vi "ExperimentCode_Serial.vi"() -> ()   [LabVIEW 2017]
uses:
  <vilib>/Analysis/baseanly.llb/Mean (DBL).vi
  <vilib>/Instr/_visa.llb/VISA Configure Serial Port (Instr).vi
  <vilib>/express/express shared/transition.llb/Dynamic To Waveform Array.vi
  <vilib>/express/express signal manip/GetorSetDDTAttributes/Set DDT Attributes/SetT0.vi
  <vilib>/express/express shared/transition.llb/Waveform Array To Dynamic.vi
  <vilib>/express/express signal manip/GetorSetDDTAttributes/Set DDT Attributes/Set DDT Properties.xnode
  <vilib>/Analysis/NI_AALBase.lvlib
panel:
  in  "Tab Control":enum32{"Setup ", "Experiment Controls", "Debug"}(tab)=enum."Experiment Controls"
  in  "Max Torque":dbl=21.3
  in  "Servo 1 Zero Offset":dbl=-4.0
  in  "Servo 2 Zero Offset":dbl=1.0
  in  "Servo 3 Zero Offset":dbl=7.0
  in  "Servo 4 Zero Offset":dbl
  in  "Servo 5 Zero Offset":dbl
  in  "Servo 5 Torque Intercept":dbl
  in  "Servo 5 Torque Slope":dbl=1.0
  in  "Servo 5 Position Intercept":dbl
  in  "Servo 5 Position Slope":dbl=1.0
  in  "Servo 4 Torque Intercept":dbl
  in  "Servo 4 Torque Slope":dbl=1.0
  in  "Servo 4 Position Intercept":dbl
  in  "Servo 4 Position Slope":dbl=1.0
  in  "Servo 3 Torque Intercept":dbl=-72.1928
  in  "Servo 3 Torque Slope":dbl=0.002332
  in  "Servo 3 Position Intercept":dbl=111.82
  in  "Servo 3 Position Slope":dbl=-0.00449
  in  "Servo 2 Torque Intercept":dbl=-72.1928
  in  "Servo 2 Torque Slope":dbl=0.002332
  in  "Servo 2 Position Intercept":dbl=97.9723
  in  "Servo 2 Position Slope":dbl=-0.00488
  in  "Servo 1 Torque Intercept":dbl=-72.1928
  in  "Servo 1 Torque Slope":dbl=0.002332
  in  "Servo 1 Position Intercept":dbl
  in  "Servo 1 Position Slope":dbl=-0.004988
  in  "Plot Last x Seconds":dbl=100.0
  in  "COM Port":refnum<visa-resource-name>
  in  "Buad Rate":i32(ring)=115200 items=["2400"=2400, "4800"=4800, "9600"=9600, "14400"=14400, "19200"=19200, "28800"=28800, "38400"=38400, "57600"=57600, "115200"=115200]
  in  "Lowest Servo Angle":dbl=-65.0
  in  "Highest Servo Angle":dbl=65.0
  in  "Number of Servos":dbl=3.0
  out "Maximum Torque Exceeded":bool
  in  "Save":bool
  in  "Stop VI":bool
  in  "Sample Frequency":dbl=100.0 step=50.0
  out "Servo Torque":cluster{" Time Offset":dbl, dbl, dbl[][]}(graph)
  in  "Tail Amplitude (cm)":dbl=2.0
  in  "Length of Segments":dbl=10.0
  in  "Number of Waves":dbl=1.0
  in  "Wave Exponential":dbl=2.0
  in  "Frequency":dbl=1.0
  in  "Wave Form":u16(ring) items=["Sine", "Exponentional Sine", "Second Mode Bending", "Flat Plate"]
  in  "Wind Up Waveform":bool
  in  "Mode 1 Amplitude":dbl=0.1 step=0.1
  in  "Mode 2 Amplitude":dbl=0.2 step=0.1
  in  "Mode 1 Phase":dbl step=0.1
  in  "Mode 2 Phase":dbl=0.8499 step=0.1
  in  "Wind Down Waveform":bool
  in  "Wind Down Time":i32=5
  out "Waveform":cluster{"X Nodes":dbl[], "Y Nodes":dbl[]}[](graph)
  in  "Servo Input":bool
  in  "Send Waveform to MBE":bool
  in  "Servo 5 Input":dbl
  in  "Servo 4 Input":dbl
  in  "Servo 3 Input":dbl
  in  "Servo 2 Input":dbl
  in  "Servo 1  Input":dbl
  out "Minimum or Maximum Angle Exceeded":bool
  in  "Filename":path=path "test.tdms"
  in  "Comment":string
  out "Calculated Sample Frequency":dbl
  out "Specified Time Delay":dbl
  out "Calculated Time Delay":dbl
  out "Time Elapsed":dbl
  out "Output Angles":dbl[](array[numeric])
  out "Input Angles":dbl[](array[numeric])
  out "Pos5 number":dbl
  out "Pos4 number":dbl
  out "Pos3 number":dbl
  out "Pos2 number":dbl
  out "Pos1 number":dbl
  out "Torq1 number":dbl
  out "Torq2 number":dbl
  out "Torq3 number":dbl
  out "Torq4 number":dbl
  out "Torq5 number":dbl
  out "Servo 1 Position":cluster{" Time Offset":dbl, "mean":dbl, dbl[][]}(graph)
  out "Servo 2 Position":cluster{" Time Offset":dbl, "mean":dbl, dbl[][]}(graph)
  out "Servo 3 Position":cluster{" Time Offset":dbl, "mean":dbl, dbl[][]}(graph)
  out "Servo 4 Position":cluster{" Time Offset":dbl, "mean":dbl, dbl[][]}(graph)
  out "Servo 5 Position":cluster{" Time Offset":dbl, "mean":dbl, dbl[][]}(graph)
  out "Sent to Arduino":string
  out "Bytes at port":cluster{i32, dbl, dbl[]}(graph)
  out "Read Buffer":string
  # "deg"
  # "deg"
  # "deg"
  # "deg"
  # "deg"
  # "Waveform"
  # "Manual"
  # "cm"
  # "Hz"
  # "Off"
  # "On"
  # "rad"
  # "rad"
  # "Off"
  # "On"
  # "Hz"
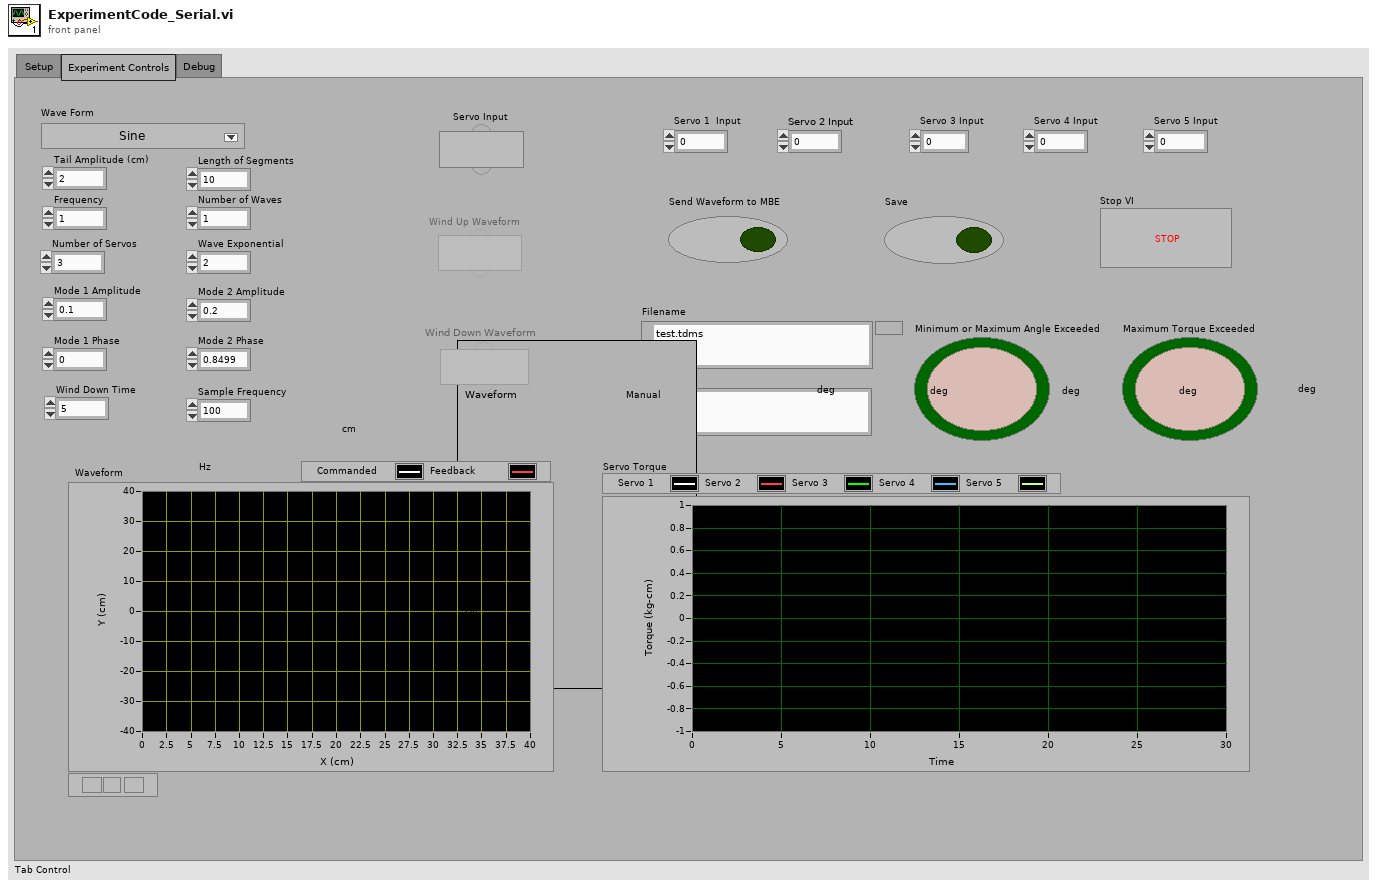
[diagram p1: front panel]
types:
  T1 = enum8{"Enabled", "Disabled", "Disabled and Grayed Out"}
  T2 = cluster{"Tail Amplitude (cm)":dbl, "Frequency":dbl, "Number of Waves":dbl, "Length of Segments":dbl, "Wave Exponential":dbl, "Number of Servos":dbl, "Mode 1 Amplitude":dbl, "Mode 2 Amplitude":dbl, "Mode 1 Phase":dbl, "Mode 2 Phase":dbl}
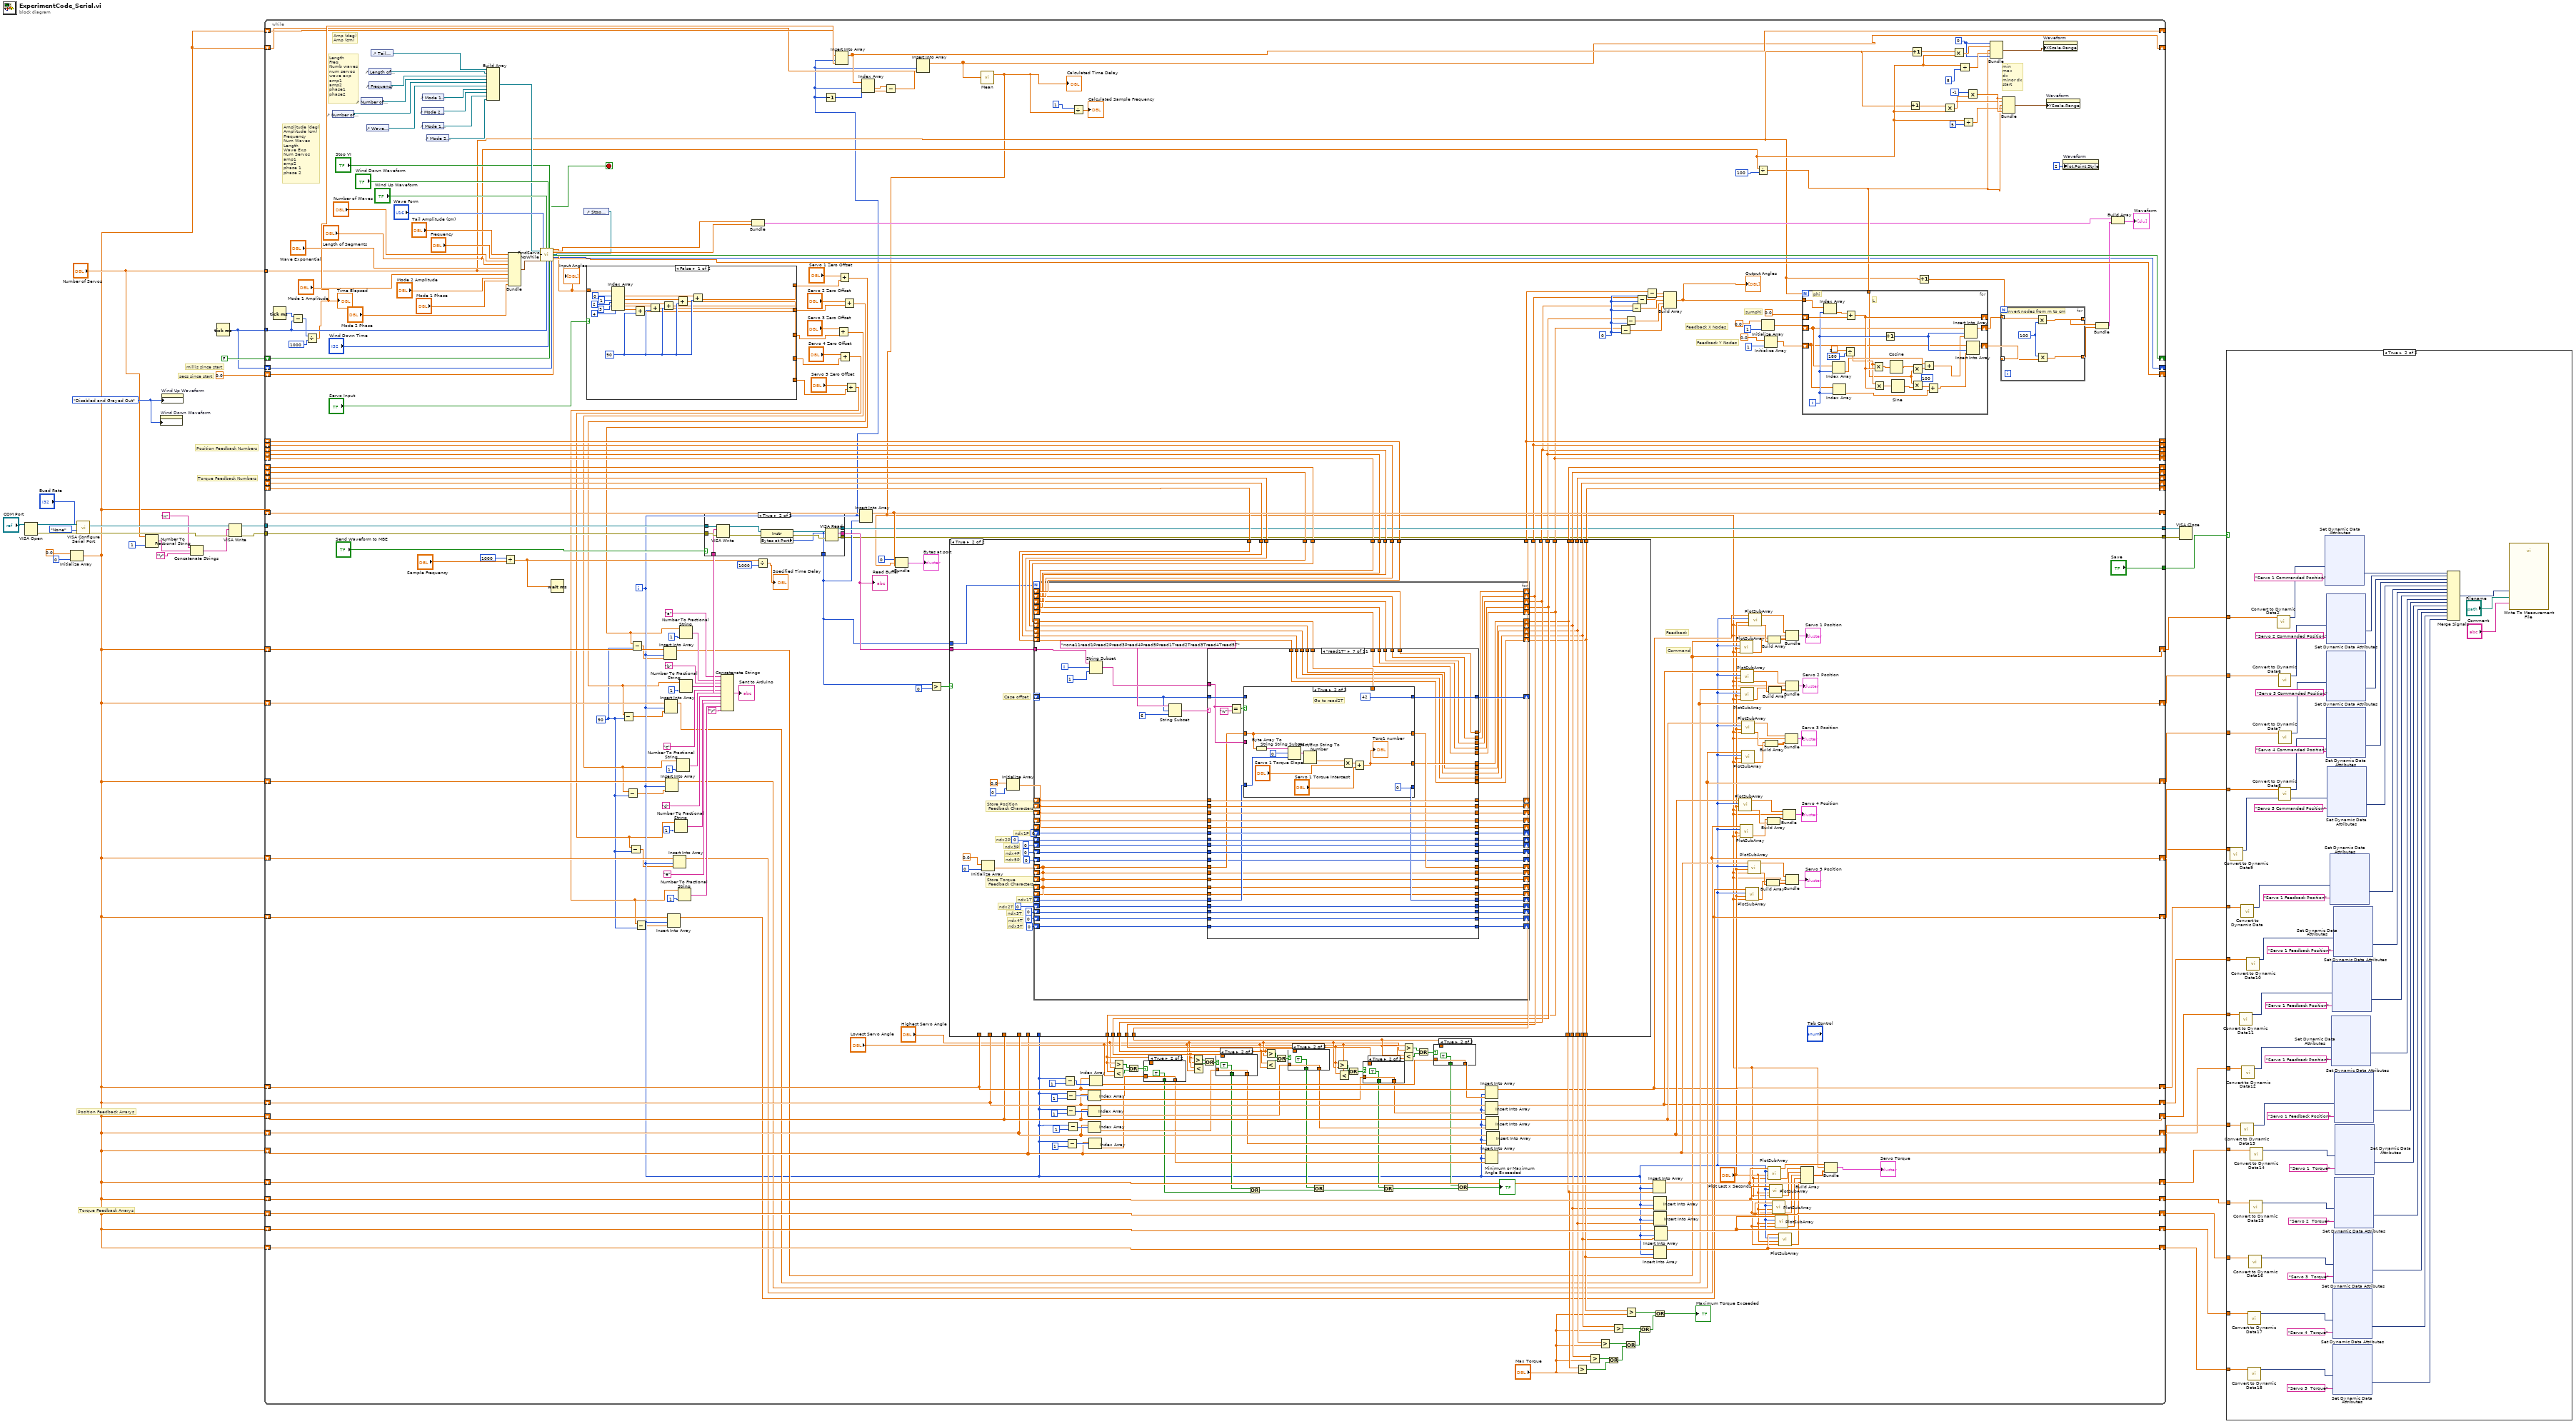
[diagram p0: block diagram]
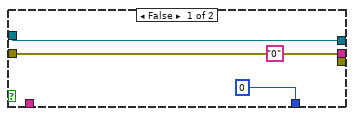
[diagram p3: hidden frame]
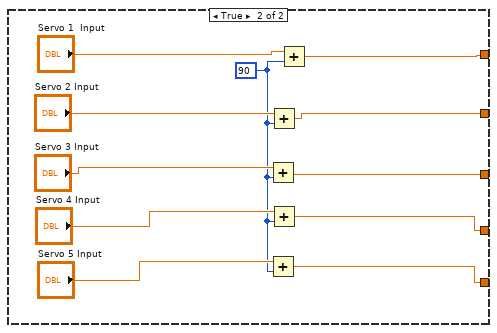
[diagram p4: hidden frame]
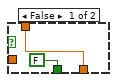
[diagram p5: hidden frame]
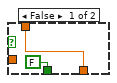
[diagram p6: hidden frame]
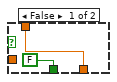
[diagram p7: hidden frame]
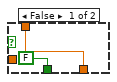
[diagram p8: hidden frame]
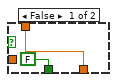
[diagram p9: hidden frame]
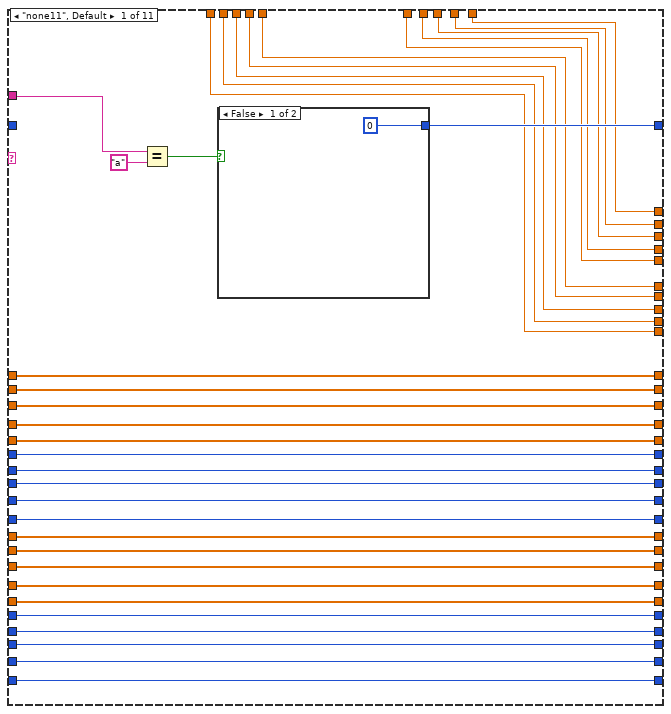
[diagram p11: hidden frame]
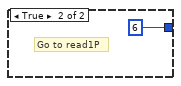
[diagram p12: hidden frame]
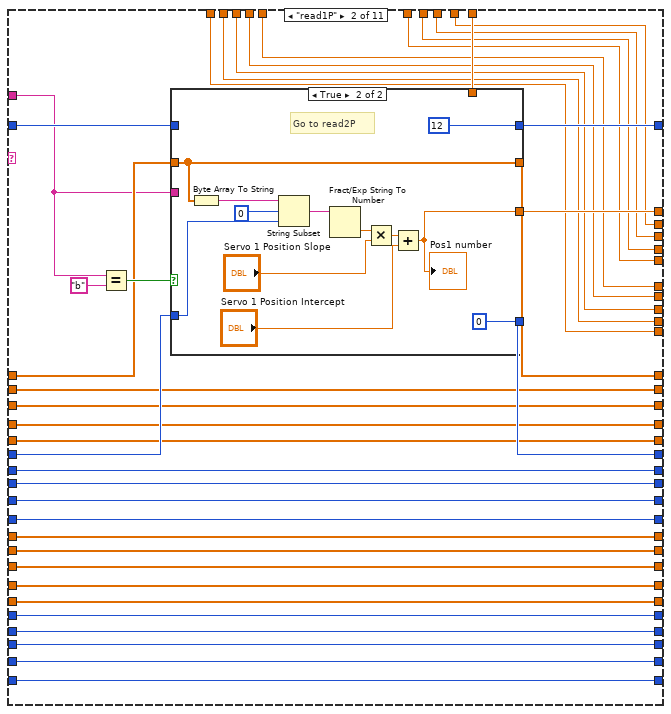
[diagram p13: hidden frame]
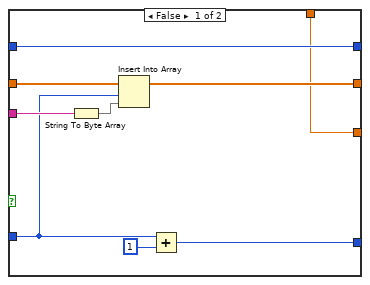
[diagram p14: hidden frame]
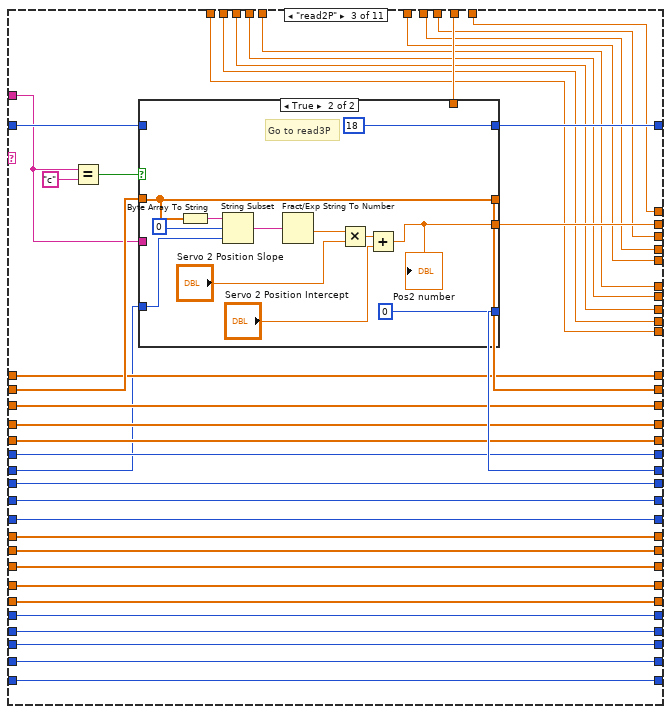
[diagram p15: hidden frame]
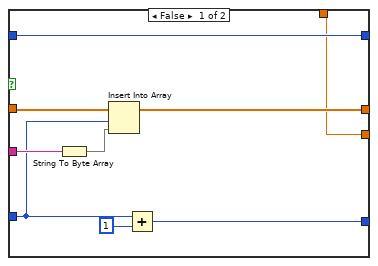
[diagram p16: hidden frame]
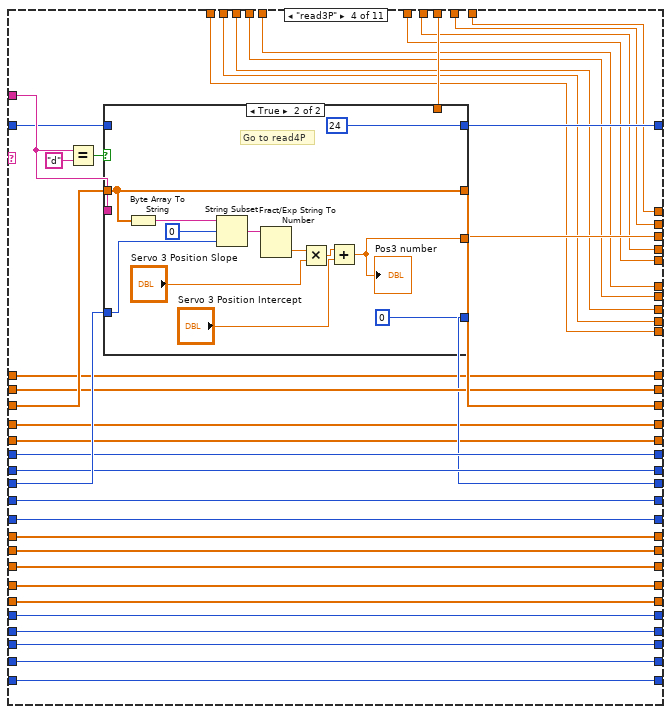
[diagram p17: hidden frame]
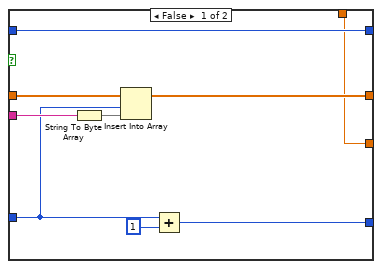
[diagram p18: hidden frame]
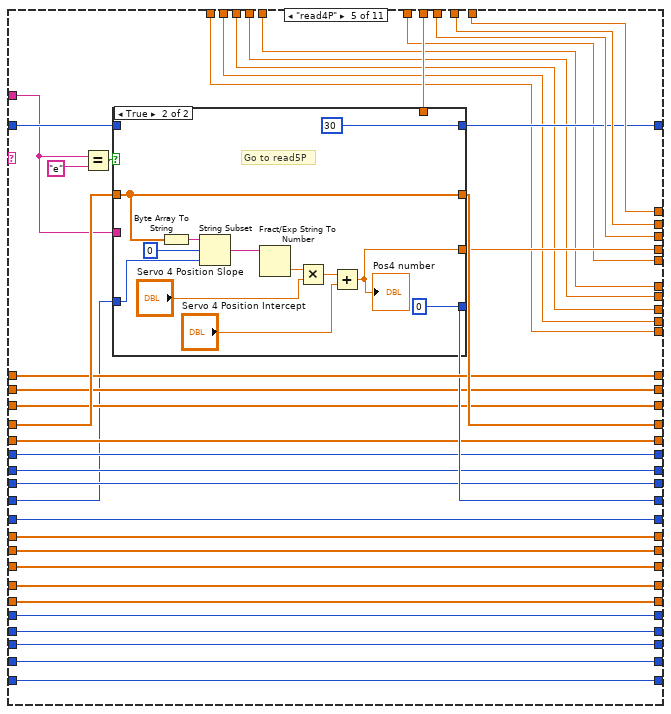
[diagram p19: hidden frame]
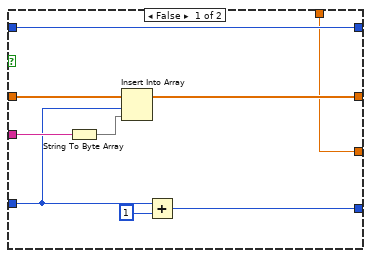
[diagram p20: hidden frame]
diagram:
  w26 = T1."Disabled and Grayed Out" ("Disabled")
  # "secs since start"
  # "millis since start"
  # "Torque Feedback Numbers"
  # "Position Feedback Numbers"
  # "Torque Feedback Arrarys"
  # "Position Feedback Arrarys"
  n1 = VISA Open(VISA resource name="COM Port") -> (VISA resource name=w37:refnum<visa-resource-name>, error out=w35:errorcluster)  [unwired: 4 in]
  n2 = Initialize Array(0.0 ("element"), 0 ("dimension size")) -> (w2:dbl[])
  n3 = call-poly "VISA Configure Serial Port"("VISA resource name"=w37, "baud rate (9600)"="Buad Rate", "parity (0:none)"=enum16{"None", "Odd", "Even", "Mark", "Space"}."None", "error in (no error)"=w35) -> ("VISA resource name out"=w12:refnum<visa-resource-name>, "error out"=w11:errorcluster)  [unwired: 10 in]
  n4 = Number To Fractional String(number="Number of Servos", precision (6)=1) -> (F-format string=w7:string)  [unwired: 2 in]
  n5 = property on="Wind Down Waveform" class="Bool (strict)"("DisabledEnum"=w26) -> ()  [unwired: 2 in, 2 out]
  n6 = property on="Wind Up Waveform" class="Bool (strict)"("DisabledEnum"=w26) -> ()  [unwired: 2 in, 2 out]
  n7 = Concatenate Strings("n", w7, "\r") -> (w3:string)
  n8 = Tick Count (ms)() -> (millisecond timer value=w32:u32)
  n9 = VISA Write(VISA resource name=w12, write buffer=w3, error in (no error)=w11) -> (VISA resource name out=w10:refnum<visa-resource-name>, error out=w9:errorcluster)  [unwired: 1 out]
  n10 = while {
    shift-right: [w340] -> _
    shift-left: w2 -> [w341]
    shift-right: [w71] -> w1
    shift-left: w2 -> [w317]
    shift-right: [w73] -> w25
    shift-left: w2 -> [w316]
    shift-right: [w77] -> w24
    shift-left: w2 -> [w315]
    shift-right: [w79] -> w23
    shift-left: w2 -> [w314]
    shift-right: [w87] -> w22
    shift-left: w2 -> [w313]
    shift-right: [w70] -> w27
    shift-left: w2 -> [w281]
    shift-right: [w72] -> w21
    shift-left: w2 -> [w273]
    shift-right: [w76] -> w20
    shift-left: w2 -> [w270]
    shift-right: [w80] -> w19
    shift-left: w2 -> [w267]
    shift-right: [w86] -> w18
    shift-left: w2 -> [w237]
    shift-right: [w140] -> _
    shift-left: _ -> [w284]
    shift-right: [w139] -> _
    shift-left: _ -> [w303]
    shift-right: [w136] -> _
    shift-left: _ -> [w306]
    shift-right: [w138] -> _
    shift-left: _ -> [w305]
    shift-right: [w137] -> _
    shift-left: _ -> [w304]
    shift-right: [w297] -> _
    shift-left: _ -> [w298]
    shift-right: [w296] -> _
    shift-left: _ -> [w299]
    shift-right: [w295] -> _
    shift-left: _ -> [w300]
    shift-right: [w294] -> _
    shift-left: _ -> [w301]
    shift-right: [w293] -> _
    shift-left: _ -> [w302]
    shift-right: [w181] -> w17
    shift-left: w2 -> [w292]
    shift-right: [w179] -> w16
    shift-left: w2 -> [w291]
    shift-right: [w178] -> w15
    shift-left: w2 -> [w290]
    shift-right: [w177] -> w14
    shift-left: w2 -> [w289]
    shift-right: [w180] -> w13
    shift-left: w2 -> [w288]
    tunnel: w9 -> [w236]
    tunnel: w32 -> [w104]
    shift-right: [w230] -> _
    shift-left: FALSE -> [w225]
    shift-right: [w94] -> _
    shift-left: w32 -> [w100]
    shift-right: [w229] -> _
    shift-left: 0.0 ("S since stop Shift Out") -> [w101]
    tunnel: ["Save"] -> w30
    tunnel: w10 -> [w235]
    tunnel: [w285] -> w29
    tunnel: [w109] -> w28
    shift-right: [w91] -> _
    shift-left: w2 -> [w98]
    tunnel: "Number of Servos" -> [w93]
    shift-right: [w88] -> _
    shift-left: w2 -> [w89]
    i -> [w68]
    stop <- w191 stop-if-true
    w45 = 90
    w125 = 0
    w141 = 0
    # "min\nmax\ndx\nminor dx\nstart"
    # "Feedback Y Nodes"
    # "Feedback X Nodes"
    # "sumphi"
    # "Command"
    # "Feedback"
    # "Amplitude (deg)\nAmplitude (cm)\nFrequency\nNum Waves\nLength\nWave Exp\nNum Servos\namp1\namp2\nphase 1\nphase 2"
    # "Amp (deg)\nAmp (cm)"
    # "Length\nFreq\nNumb waves\nnum servos\nwave exp\namp1\namp2\nphase1\nphase2"
    n11 = Tick Count (ms)() -> (millisecond timer value=w105:u32)
    n12 = Subtract(x=w105, y=w104) -> (x-y=w103:u32)
    n13 = Divide(x=w103, y=1000) -> (x/y=w99:dbl)
    "Time Elapsed" <- w99
    n14 = control-ref of="Number of Servos"() -> (w92:refnum<vi>)
    n15 = control-ref of="Number of Waves"() -> (w210:refnum<vi>)
    n16 = control-ref of="Wave Exponential"() -> (w209:refnum<vi>)
    n17 = control-ref of="Length of Segments"() -> (w212:refnum<vi>)
    n18 = control-ref of="Frequency"() -> (w211:refnum<vi>)
    n19 = control-ref of="Tail Amplitude (cm)"() -> (w195:refnum<vi>)
    n20 = control-ref of="Mode 2 Amplitude"() -> (w207:refnum<vi>)
    n21 = control-ref of="Mode 1 Amplitude"() -> (w208:refnum<vi>)
    n22 = control-ref of="Mode 1 Phase"() -> (w206:refnum<vi>)
    n23 = control-ref of="Mode 2 Phase"() -> (w205:refnum<vi>)
    n24 = Build Array(w195, w212, w211, w210, w92, w209, w208, w207, w206, w205) -> (w196:refnum<vi>[])
    n25 = Divide(x=1000, y="Sample Frequency") -> (x/y=w107:dbl)
    n26 = Bundle("Tail Amplitude (cm)"="Tail Amplitude (cm)", "Frequency"="Frequency", "Number of Waves"="Number of Waves", "Length of Segments"="Length of Segments", "Wave Exponential"="Wave Exponential", "Number of Servos"=w93, "Mode 1 Amplitude"="Mode 1 Amplitude", "Mode 2 Amplitude"="Mode 2 Amplitude", "Mode 1 Phase"="Mode 1 Phase", "Mode 2 Phase"="Mode 2 Phase") -> (w41:T2)  [unwired: 1 in]
    n27 = Wait (ms)(milliseconds to wait=w107) -> ()  [unwired: 1 out]
    n28 = control-ref of="Stop Reference"() -> (w224:refnum<vi>)
    n29 = call "FindServo_NoWhile.vi"("Parameter Reference Arrary"=w196, "Parameter Cluster"=w41, "Wave Form"="Wave Form", "Wind Up"="Wind Up Waveform", "Start Time (Tick Count-millis)"=w104, "Wind Down"="Wind Down Waveform", "Wind Down Time"="Wind Down Time", "Stop In"="Stop VI", "Stop Pressed Shift In (False)"=w225, "Ms Since Stop Shift In (Start Time)"=w100, "Stop In Reference"=w224, "S since stop Shift In"=w101) -> ("Stop Out"=w191:bool, "phi"=w110:dbl[], "X Nodes"=w228:dbl[], "Y Nodes"=w227:dbl[], "Stop Pressed Shift Out (False)"=w230:bool, "MS Since Stop Shift Out"=w94:u32, "S since stop Shift Out"=w229:dbl)  [unwired: 9 in]
    "Input Angles" <- w110
    n30 = case shown="False" "Servo Input" {
      tunnel: [w390 w413] -> w218
      tunnel: [w389 w405] -> w217
      tunnel: [w388 w404] -> w216
      tunnel: [w387 w409] -> w215
      tunnel: [w386 w410] -> w214
      tunnel: w110 -> [w402 _]
      frame False {
        w391 = 90
        n31 = Index Array(array=w402, index #1=0, index #2=1, index #3=2, index #4=3, index #5=4) -> (element #1=w396:dbl, element #2=w395:dbl, element #3=w394:dbl, element #4=w393:dbl, element #5=w392:dbl)
        n32 = Add(x=w392, y=w391) -> (x+y=w386:dbl)
        n33 = Add(x=w393, y=w391) -> (x+y=w387:dbl)
        n34 = Add(x=w394, y=w391) -> (x+y=w388:dbl)
        n35 = Add(x=w395, y=w391) -> (x+y=w389:dbl)
        n36 = Add(x=w396, y=w391) -> (x+y=w390:dbl)
      }
      frame True {
        w403 = 90
        n37 = Add(x="Servo 3 Input", y=w403) -> (x+y=w404:dbl)
        n38 = Add(x="Servo 5 Input", y=w403) -> (x+y=w410:dbl)
        n39 = Add(x="Servo 2 Input", y=w403) -> (x+y=w405:dbl)
        n40 = Add(x="Servo 4 Input", y=w403) -> (x+y=w409:dbl)
        n41 = Add(x="Servo 1  Input", y=w403) -> (x+y=w413:dbl)
      }
    }
    n42 = Bundle("X Nodes"=w228, "Y Nodes"=w227) -> (w120:cluster{"X Nodes":dbl[], "Y Nodes":dbl[]})  [unwired: 1 in]
    n43 = Divide(x=w107, y=1000) -> (x/y=→"Specified Time Delay":dbl)
    n44 = Decrement(x=w68) -> (x-1=w95:i32)
    n45 = Insert Into Array(array=w98, index=w68, new element=w99) -> (w91:dbl[])
    n46 = Add(x="Servo 3 Zero Offset", y=w216) -> (x+y=w50:dbl)
    n47 = Subtract(x=w50, y=w45) -> (x-y=w51:dbl)
    n48 = Insert Into Array(array=w315, index=w68, new element=w51) -> (w77:dbl[])
    n49 = Number To Fractional String(number=w50, precision (6)=1) -> (F-format string=w336:string)  [unwired: 2 in]
    n50 = Add(x="Servo 1 Zero Offset", y=w218) -> (x+y=w54:dbl)
    n51 = Subtract(x=w54, y=w45) -> (x-y=w55:dbl)
    n52 = Insert Into Array(array=w317, index=w68, new element=w55) -> (w71:dbl[])
    n53 = Number To Fractional String(number=w54, precision (6)=1) -> (F-format string=w338:string)  [unwired: 2 in]
    n54 = Add(x="Servo 4 Zero Offset", y=w215) -> (x+y=w48:dbl)
    n55 = Subtract(x=w48, y=w45) -> (x-y=w49:dbl)
    n56 = Insert Into Array(array=w314, index=w68, new element=w49) -> (w79:dbl[])
    n57 = Number To Fractional String(number=w48, precision (6)=1) -> (F-format string=w329:string)  [unwired: 2 in]
    n58 = Add(x="Servo 2 Zero Offset", y=w217) -> (x+y=w52:dbl)
    n59 = Subtract(x=w52, y=w45) -> (x-y=w53:dbl)
    n60 = Insert Into Array(array=w316, index=w68, new element=w53) -> (w73:dbl[])
    n61 = Number To Fractional String(number=w52, precision (6)=1) -> (F-format string=w337:string)  [unwired: 2 in]
    n62 = Add(x="Servo 5 Zero Offset", y=w214) -> (x+y=w46:dbl)
    n63 = Subtract(x=w46, y=w45) -> (x-y=w47:dbl)
    n64 = Insert Into Array(array=w313, index=w68, new element=w47) -> (w87:dbl[])
    n65 = Number To Fractional String(number=w46, precision (6)=1) -> (F-format string=w328:string)  [unwired: 2 in]
    n66 = Concatenate Strings("a", w338, "b", w337, "c", w336, "d", w329, "e", w328, "\r") -> (w339:string)
    "Sent to Arduino" <- w339
    n67 = case shown="True" "Send Waveform to MBE" {
      tunnel: w339 -> [_ w375]
      tunnel: ["0" w385] -> w324
      tunnel: [w373 w384] -> w109
      tunnel: [w374 w383] -> w285
      tunnel: [0 w378] -> w194
      tunnel: w236 -> [w373 w377]
      tunnel: w235 -> [w374 w376]
      frame False {
      }
      frame True {
        n68 = VISA Write(VISA resource name=w376, write buffer=w375, error in (no error)=w377) -> (VISA resource name out=w382:refnum<visa-resource-name>, error out=w379:errorcluster)  [unwired: 1 out]
        n69 = property class="Instr"(reference=w382, error in=w379) -> (reference out=w381:refnum<visa-resource-name>, error out=w380:errorcluster, "Bytes at Port"=w378:u32)
        n70 = VISA Read(VISA resource name=w381, byte count=w378, error in (no error)=w380) -> (VISA resource name out=w383:refnum<visa-resource-name>, read buffer=w385:string, error out=w384:errorcluster)  [unwired: 1 out]
      }
    }
    "Read Buffer" <- w324
    n71 = Insert Into Array(array=w341, index=w68, new element=w194) -> (w340:dbl[])
    n72 = Index Array(array=w91, index #1=w68, index #2=w95) -> (element #1=w97:dbl, element #2=w96:dbl)
    n73 = Subtract(x=w97, y=w96) -> (x-y=w90:dbl)
    n74 = Insert Into Array(array=w89, index=w68, new element=w90) -> (w88:dbl[])
    n75 = Greater?(x=w194, y=0) -> (0:w287:bool)
    n76 = case shown="True" w287 {
      tunnel: w194 -> [_ w444]
      tunnel: w324 -> [_ w482]
      tunnel: [w443 w456] -> w276
      tunnel: w68 -> [_ _]
      tunnel: w281 -> [_ _]
      tunnel: [w442 w455] -> w258
      tunnel: [w441 w454] -> w252
      tunnel: [w440 w453] -> w246
      tunnel: [w439 w452] -> w242
      tunnel: w273 -> [_ _]
      tunnel: w270 -> [_ _]
      tunnel: w267 -> [_ _]
      tunnel: w237 -> [_ _]
      tunnel: w284 -> [w443 w473]
      tunnel: w303 -> [w442 w472]
      tunnel: w306 -> [w441 w471]
      tunnel: w305 -> [w440 w470]
      tunnel: w304 -> [w439 w469]
      tunnel: [w443 w456] -> w140
      tunnel: [w442 w455] -> w139
      tunnel: [w441 w454] -> w136
      tunnel: [w440 w453] -> w138
      tunnel: [w439 w452] -> w137
      tunnel: w302 -> [w434 w446]
      tunnel: w301 -> [w435 w448]
      tunnel: w300 -> [w436 w468]
      tunnel: w299 -> [w437 w467]
      tunnel: w298 -> [w438 w466]
      tunnel: [w438 w451] -> w297
      tunnel: [w437 w450] -> w296
      tunnel: [w436 w449] -> w295
      tunnel: [w435 w447] -> w294
      tunnel: [w434 w445] -> w293
      tunnel: [w438 w451] -> w169
      tunnel: [w437 w450] -> w165
      tunnel: [w436 w449] -> w166
      tunnel: [w435 w447] -> w167
      tunnel: [w434 w445] -> w168
      frame False {
      }
      frame True {
        # "Store Torque\n Feedback Characters"
        # "ndx5T"
        # "ndx4T"
        # "ndx3T"
        # "ndx2T"
        # "ndx1T"
        # "Store Position\n Feedback Characters"
        # "ndx5P"
        # "ndx4P"
        # "ndx3P"
        # "ndx2P"
        # "ndx1P"
        # "Case offset"
        n77 = Initialize Array(0.0 ("element"), 0 ("dimension size")) -> (w463:dbl[])
        n78 = Initialize Array(0.0 ("element"), 0 ("dimension size")) -> (w476:dbl[])
        n79 = for {
          N: w444 -> [_]
          tunnel: w482 -> [w550]
          shift-right: [w548] -> _
          shift-left: 1 -> [w493]
          shift-right: [w547] -> _
          shift-left: 0 -> [w546]
          shift-right: [w544] -> _
          shift-left: w476 -> [w545]
          shift-right: [w542] -> _
          shift-left: w476 -> [w543]
          shift-right: [w538] -> _
          shift-left: 0 -> [w541]
          shift-right: [w539] -> _
          shift-left: 0 -> [w540]
          shift-right: [w536] -> _
          shift-left: w476 -> [w537]
          shift-right: [w528] -> _
          shift-left: w476 -> [w535]
          shift-right: [w529] -> _
          shift-left: w476 -> [w534]
          shift-right: [w532] -> _
          shift-left: 0 -> [w533]
          shift-right: [w530] -> _
          shift-left: 0 -> [w531]
          shift-right: [w515] -> _
          shift-left: w463 -> [w516]
          shift-right: [w514] -> _
          shift-left: w463 -> [w513]
          shift-right: [w512] -> _
          shift-left: w463 -> [w511]
          shift-right: [w510] -> _
          shift-left: w463 -> [w509]
          shift-right: [w508] -> _
          shift-left: w463 -> [w507]
          shift-right: [w506] -> _
          shift-left: 0 -> [w505]
          shift-right: [w504] -> _
          shift-left: 0 -> [w503]
          shift-right: [w502] -> _
          shift-left: 0 -> [w501]
          shift-right: [w499] -> _
          shift-left: 0 -> [w500]
          shift-right: [w498] -> _
          shift-left: 0 -> [w497]
          shift-right: [w492] -> w456
          shift-left: w473 -> [w523]
          shift-right: [w491] -> w455
          shift-left: w472 -> [w527]
          shift-right: [w490] -> w454
          shift-left: w471 -> [w526]
          shift-right: [w489] -> w453
          shift-left: w470 -> [w525]
          shift-right: [w488] -> w452
          shift-left: w469 -> [w524]
          shift-right: [w487] -> w451
          shift-left: w466 -> [w517]
          shift-right: [w486] -> w450
          shift-left: w467 -> [w518]
          shift-right: [w485] -> w449
          shift-left: w468 -> [w519]
          shift-right: [w484] -> w447
          shift-left: w448 -> [w520]
          shift-right: [w483] -> w445
          shift-left: w446 -> [w521]
          i -> [w494]
          n80 = String Subset(string=w550, offset (0)=w494, length (rest)=1 ("length (rest)")) -> (substring=w522:string)
          n81 = String Subset(string="none11read1Pread2Pread3Pread4Pread5Pread1Tread2Tread3Tread4Tread5T", offset (0)=w493, length (rest)=6 ("length (rest)")) -> (substring=w496:string)
          n82 = case shown="\"read1T\"" w496 {
            tunnel: w522 -> [w585 w619 w675 w729 w796 w855 w916 w975 w1034 w1093 w1152]
            tunnel: [w582 w622 w677 w736 w782 w858 w919 w978 w1037 w1096 w1155] -> w548
            tunnel: [w581 w617 w679 w741 w794 w848 w911 w970 w1029 w1088 w1147] -> w547
            tunnel: w546 -> [w581 w618 w679 w741 w794 w848 w911 w970 w1029 w1088 w1147]
            tunnel: w545 -> [w578 w620 w674 w724 w800 w852 w915 w974 w1033 w1092 w1151]
            tunnel: [w578 w623 w674 w724 w800 w852 w915 w974 w1033 w1092 w1151] -> w544
            tunnel: w543 -> [w579 w616 w684 w737 w792 w851 w914 w973 w1032 w1091 w1150]
            tunnel: [w579 w616 w683 w737 w792 w851 w914 w973 w1032 w1091 w1150] -> w542
            tunnel: w541 -> [w580 w612 w662 w740 w793 w847 w910 w969 w1028 w1087 w1146]
            tunnel: [w580 w612 w682 w740 w793 w847 w910 w969 w1028 w1087 w1146] -> w538
            tunnel: w493 -> [_ w621 w678 w721 w797 w857 w918 w977 w1036 w1095 w1154]
            tunnel: w540 -> [w575 w611 w676 w742 w789 w846 w909 w968 w1027 w1086 w1145]
            tunnel: [w575 w611 w676 w733 w789 w846 w909 w968 w1027 w1086 w1145] -> w539
            tunnel: w537 -> [w572 w615 w673 w739 w791 w850 w913 w972 w1031 w1090 w1149]
            tunnel: [w572 w615 w673 w738 w791 w850 w913 w972 w1031 w1090 w1149] -> w536
            tunnel: w535 -> [w573 w614 w672 w732 w802 w849 w912 w971 w1030 w1089 w1148]
            tunnel: w534 -> [w574 w613 w671 w731 w790 w860 w903 w962 w1014 w1073 w1132]
            tunnel: w533 -> [w577 w610 w670 w735 w781 w845 w908 w967 w1026 w1085 w1144]
            tunnel: [w577 w610 w670 w735 w795 w845 w908 w967 w1026 w1085 w1144] -> w532
            tunnel: w531 -> [w576 w609 w669 w734 w788 w854 w900 w951 w1011 w1067 w1129]
            tunnel: [w576 w609 w669 w734 w788 w853 w900 w951 w1011 w1067 w1129] -> w530
            tunnel: [w574 w613 w671 w731 w790 w859 w903 w962 w1014 w1073 w1132] -> w529
            tunnel: [w573 w614 w672 w732 w801 w849 w912 w971 w1030 w1089 w1148] -> w528
            tunnel: [w567 w608 w666 w722 w783 w844 w907 w966 w1025 w1084 w1143] -> w492
            tunnel: w523 -> [w567 w607 w666 w722 w783 w844 w907 w966 w1025 w1084 w1143]
            tunnel: [w571 w606 w668 w728 w787 w839 w904 w963 w1022 w1081 w1140] -> w491
            tunnel: w527 -> [w571 w606 w667 w728 w787 w839 w904 w963 w1022 w1081 w1140]
            tunnel: [w570 w605 w663 w727 w784 w842 w906 w965 w1024 w1083 w1142] -> w490
            tunnel: w526 -> [w570 w605 w663 w726 w784 w842 w906 w965 w1024 w1083 w1142]
            tunnel: [w569 w604 w665 w725 w786 w840 w905 w964 w1023 w1082 w1141] -> w489
            tunnel: w525 -> [w569 w604 w665 w725 w785 w840 w905 w964 w1023 w1082 w1141]
            tunnel: [w568 w603 w664 w723 w765 w843 w896 w946 w1020 w1080 w1139] -> w488
            tunnel: w524 -> [w568 w603 w664 w723 w765 w841 w896 w946 w1020 w1080 w1139]
            tunnel: w521 -> [w562 w598 w657 w716 w776 w834 w884 w942 w1015 w1074 w1138]
            tunnel: w520 -> [w563 w599 w658 w717 w777 w835 w885 w943 w1017 w1079 w1133]
            tunnel: w519 -> [w564 w600 w659 w718 w778 w836 w886 w944 w1021 w1076 w1134]
            tunnel: w518 -> [w565 w601 w660 w719 w779 w837 w887 w948 w1018 w1077 w1135]
            tunnel: w517 -> [w566 w602 w661 w720 w780 w838 w897 w947 w1019 w1078 w1136]
            tunnel: [w566 w602 w661 w720 w780 w838 w895 w947 w1019 w1078 w1136] -> w487
            tunnel: [w565 w601 w660 w719 w779 w837 w887 w945 w1018 w1077 w1135] -> w486
            tunnel: [w564 w600 w659 w718 w778 w836 w886 w944 w1016 w1076 w1134] -> w485
            tunnel: [w563 w599 w658 w717 w777 w835 w885 w943 w1017 w1075 w1133] -> w484
            tunnel: [w562 w598 w657 w716 w776 w834 w884 w942 w1015 w1074 w1137] -> w483
            tunnel: w516 -> [w561 w597 w656 w715 w775 w833 w902 w959 w1008 w1070 w1119]
            tunnel: [w561 w597 w656 w715 w775 w833 w901 w959 w1008 w1070 w1119] -> w515
            tunnel: [w560 w596 w655 w714 w774 w832 w894 w960 w1007 w1069 w1120] -> w514
            tunnel: w513 -> [w560 w596 w655 w714 w774 w832 w894 w961 w1007 w1069 w1120]
            tunnel: [w559 w595 w654 w713 w773 w831 w893 w958 w1012 w1068 w1121] -> w512
            tunnel: w511 -> [w559 w595 w654 w713 w773 w831 w893 w958 w1013 w1068 w1121]
            tunnel: [w558 w594 w653 w712 w772 w830 w892 w957 w1006 w1072 w1122] -> w510
            tunnel: w509 -> [w558 w594 w653 w712 w772 w830 w892 w957 w1006 w1071 w1122]
            tunnel: [w557 w593 w652 w711 w771 w829 w891 w956 w1005 w1063 w1131] -> w508
            tunnel: w507 -> [w557 w593 w652 w711 w771 w829 w891 w956 w1005 w1063 w1130]
            tunnel: [w556 w592 w651 w710 w770 w828 w898 w955 w1004 w1064 w1123] -> w506
            tunnel: w505 -> [w556 w592 w651 w710 w770 w828 w899 w955 w1004 w1064 w1123]
            tunnel: [w555 w591 w650 w709 w769 w827 w890 w950 w1003 w1062 w1124] -> w504
            tunnel: w503 -> [w555 w591 w650 w709 w769 w827 w890 w949 w1003 w1062 w1124]
            tunnel: [w554 w590 w649 w708 w768 w826 w889 w954 w1010 w1061 w1125] -> w502
            tunnel: w501 -> [w554 w590 w649 w708 w768 w826 w889 w954 w1009 w1061 w1125]
            tunnel: w500 -> [w553 w589 w648 w707 w767 w825 w888 w953 w1002 w1065 w1126]
            tunnel: [w553 w589 w648 w707 w767 w825 w888 w953 w1002 w1066 w1126] -> w499
            tunnel: [w552 w588 w647 w706 w766 w824 w883 w952 w1001 w1060 w1128] -> w498
            tunnel: w497 -> [w552 w588 w647 w706 w766 w824 w883 w952 w1001 w1060 w1127]
            frame "none11", Default {
              n83 = Equal?(x=w585, y="a") -> (x = y?=w583:bool)
              n84 = case shown="False" w583 {
                tunnel: [0 6] -> w582
                frame False {
                }
                frame True {
                  # "Go to read1P"
                }
              }
            }
            frame "read1P" {
              n85 = Equal?(x=w619, y="b") -> (x = y?=w624:bool)
              n86 = case shown="True" w624 {
                tunnel: [w634 0] -> w617
                tunnel: w620 -> [w628 w642]
                tunnel: [w632 w642] -> w623
                tunnel: w619 -> [w631 _]
                tunnel: [w629 12] -> w622
                tunnel: w621 -> [w629 _]
                tunnel: w618 -> [w627 w641]
                tunnel: [w626 w639] -> w608
                tunnel: w607 -> [w626 _]
                frame False {
                  n87 = String To Byte Array(string=w631) -> (unsigned byte array=w630:u8[])
                  n88 = Insert Into Array(array=w628, index=w627, new element=w630) -> (w632:dbl[])
                  n89 = Add(x=w627, y=1) -> (x+y=w634:i32)
                }
                frame True {
                  # "Go to read2P"
                  n90 = Byte Array To String(unsigned byte array=w642) -> (string=w643:string)
                  n91 = String Subset(string=w643, offset (0)=0, length (rest)=w641) -> (substring=w640:string)
                  n92 = Fract/Exp String To Number(string=w640) -> (number=w638:dbl)  [unwired: 3 in, 1 out]
                  n93 = Multiply(x=w638, y="Servo 1 Position Slope") -> (x*y=w637:dbl)
                  n94 = Add(x=w637, y="Servo 1 Position Intercept") -> (x+y=w639:dbl)
                  "Pos1 number" <- w639
                }
              }
            }
            frame "read2P" {
              n95 = Equal?(x=w675, y="c") -> (x = y?=w680:bool)
              n96 = case shown="True" w680 {
                tunnel: [w693 0] -> w682
                tunnel: w662 -> [w687 w702]
                tunnel: w684 -> [w691 w700]
                tunnel: [w690 w700] -> w683
                tunnel: w675 -> [w689 _]
                tunnel: [w686 18] -> w677
                tunnel: w678 -> [w686 _]
                tunnel: [w685 w696] -> w668
                tunnel: w667 -> [w685 _]
                frame False {
                  n97 = String To Byte Array(string=w689) -> (unsigned byte array=w688:u8[])
                  n98 = Insert Into Array(array=w691, index=w687, new element=w688) -> (w690:dbl[])
                  n99 = Add(x=w687, y=1) -> (x+y=w693:i32)
                }
                frame True {
                  # "Go to read3P"
                  n100 = Byte Array To String(unsigned byte array=w700) -> (string=w699:string)
                  n101 = String Subset(string=w699, offset (0)=0, length (rest)=w702) -> (substring=w701:string)
                  n102 = Fract/Exp String To Number(string=w701) -> (number=w697:dbl)  [unwired: 3 in, 1 out]
                  n103 = Multiply(x=w697, y="Servo 2 Position Slope") -> (x*y=w698:dbl)
                  n104 = Add(x=w698, y="Servo 2 Position Intercept") -> (x+y=w696:dbl)
                  "Pos2 number" <- w696
                }
              }
            }
            frame "read3P" {
              n105 = Equal?(x=w729, y="d") -> (x = y?=w743:bool)
              n106 = case shown="True" w743 {
                tunnel: [w752 0] -> w733
                tunnel: w742 -> [w746 w759]
                tunnel: w739 -> [w750 w760]
                tunnel: [w749 w760] -> w738
                tunnel: w729 -> [w748 _]
                tunnel: [w745 24] -> w736
                tunnel: w721 -> [w745 _]
                tunnel: [w744 w753] -> w727
                tunnel: w726 -> [w744 _]
                frame False {
                  n107 = String To Byte Array(string=w748) -> (unsigned byte array=w747:u8[])
                  n108 = Insert Into Array(array=w750, index=w746, new element=w747) -> (w749:dbl[])
                  n109 = Add(x=w746, y=1) -> (x+y=w752:i32)
                }
                frame True {
                  # "Go to read4P"
                  n110 = Byte Array To String(unsigned byte array=w760) -> (string=w761:string)
                  n111 = String Subset(string=w761, offset (0)=0, length (rest)=w759) -> (substring=w758:string)
                  n112 = Fract/Exp String To Number(string=w758) -> (number=w756:dbl)  [unwired: 3 in, 1 out]
                  n113 = Multiply(x=w756, y="Servo 3 Position Slope") -> (x*y=w757:dbl)
                  n114 = Add(x=w757, y="Servo 3 Position Intercept") -> (x+y=w753:dbl)
                  "Pos3 number" <- w753
                }
              }
            }
            frame "read4P" {
              n115 = Equal?(x=w796, y="e") -> (x = y?=w798:bool)
              n116 = case shown="True" w798 {
                tunnel: [w811 0] -> w795
                tunnel: w781 -> [w805 w819]
                tunnel: w802 -> [w809 w820]
                tunnel: [w808 w820] -> w801
                tunnel: w796 -> [w807 _]
                tunnel: [w804 30] -> w782
                tunnel: w797 -> [w804 _]
                tunnel: [w803 w816] -> w786
                tunnel: w785 -> [w803 _]
                frame False {
                  n117 = String To Byte Array(string=w807) -> (unsigned byte array=w806:u8[])
                  n118 = Insert Into Array(array=w809, index=w805, new element=w806) -> (w808:dbl[])
                  n119 = Add(x=w805, y=1) -> (x+y=w811:i32)
                }
                frame True {
                  # "Go to read5P"
                  n120 = Byte Array To String(unsigned byte array=w820) -> (string=w821:string)
                  n121 = String Subset(string=w821, offset (0)=0, length (rest)=w819) -> (substring=w818:string)
                  n122 = Fract/Exp String To Number(string=w818) -> (number=w815:dbl)  [unwired: 3 in, 1 out]
                  n123 = Multiply(x=w815, y="Servo 4 Position Slope") -> (x*y=w817:dbl)
                  n124 = Add(x=w817, y="Servo 4 Position Intercept") -> (x+y=w816:dbl)
                  "Pos4 number" <- w816
                }
              }
            }
            frame "read5P" {
              n125 = Equal?(x=w855, y="v") -> (x = y?=w856:bool)
              n126 = case shown="True" w856 {
                tunnel: [w870 0] -> w853
                tunnel: w854 -> [w864 w877]
                tunnel: w860 -> [w868 w878]
                tunnel: [w867 w878] -> w859
                tunnel: w855 -> [w866 _]
                tunnel: [w863 36] -> w858
                tunnel: w857 -> [w863 _]
                tunnel: [w862 w872] -> w843
                tunnel: w841 -> [w862 _]
                frame False {
                  n127 = String To Byte Array(string=w866) -> (unsigned byte array=w865:u8[])
                  n128 = Insert Into Array(array=w868, index=w864, new element=w865) -> (w867:dbl[])
                  n129 = Add(x=w864, y=1) -> (x+y=w870:i32)
                }
                frame True {
                  # "Go to read1T"
                  n130 = Byte Array To String(unsigned byte array=w878) -> (string=w879:string)
                  n131 = String Subset(string=w879, offset (0)=0, length (rest)=w877) -> (substring=w876:string)
                  n132 = Fract/Exp String To Number(string=w876) -> (number=w874:dbl)  [unwired: 3 in, 1 out]
                  n133 = Multiply(x=w874, y="Servo 5 Position Slope") -> (x*y=w875:dbl)
                  n134 = Add(x=w875, y="Servo 5 Position Intercept") -> (x+y=w872:dbl)
                  "Pos5 number" <- w872
                }
              }
            }
            frame "read1T" {
              n135 = Equal?(x=w916, y="w") -> (x = y?=w917:bool)
              n136 = case shown="True" w917 {
                tunnel: [w929 0] -> w898
                tunnel: w899 -> [w923 w935]
                tunnel: w902 -> [w927 w937]
                tunnel: [w926 w937] -> w901
                tunnel: w916 -> [w925 _]
                tunnel: [w922 42] -> w919
                tunnel: w918 -> [w922 _]
                tunnel: [w921 w932] -> w895
                tunnel: w897 -> [w921 _]
                frame False {
                  n137 = String To Byte Array(string=w925) -> (unsigned byte array=w924:u8[])
                  n138 = Insert Into Array(array=w927, index=w923, new element=w924) -> (w926:dbl[])
                  n139 = Add(x=w923, y=1) -> (x+y=w929:i32)
                }
                frame True {
                  # "Go to read2T"
                  n140 = Byte Array To String(unsigned byte array=w937) -> (string=w938:string)
                  n141 = String Subset(string=w938, offset (0)=0, length (rest)=w935) -> (substring=w936:string)
                  n142 = Fract/Exp String To Number(string=w936) -> (number=w933:dbl)  [unwired: 3 in, 1 out]
                  n143 = Multiply(x=w933, y="Servo 1 Torque Slope") -> (x*y=w934:dbl)
                  n144 = Add(x=w934, y="Servo 1 Torque Intercept") -> (x+y=w932:dbl)
                  "Torq1 number" <- w932
                }
              }
            }
            frame "read2T" {
              n145 = Equal?(x=w975, y="x") -> (x = y?=w976:bool)
              n146 = case shown="True" w976 {
                tunnel: [w988 0] -> w950
                tunnel: w949 -> [w982 w994]
                tunnel: w961 -> [w986 w996]
                tunnel: [w985 w996] -> w960
                tunnel: w975 -> [w984 _]
                tunnel: [w981 48] -> w978
                tunnel: w977 -> [w981 _]
                tunnel: [w980 w991] -> w945
                tunnel: w948 -> [w980 _]
                frame False {
                  n147 = String To Byte Array(string=w984) -> (unsigned byte array=w983:u8[])
                  n148 = Insert Into Array(array=w986, index=w982, new element=w983) -> (w985:dbl[])
                  n149 = Add(x=w982, y=1) -> (x+y=w988:i32)
                }
                frame True {
                  # "Go to read3T"
                  n150 = Byte Array To String(unsigned byte array=w996) -> (string=w997:string)
                  n151 = String Subset(string=w997, offset (0)=0, length (rest)=w994) -> (substring=w995:string)
                  n152 = Fract/Exp String To Number(string=w995) -> (number=w992:dbl)  [unwired: 3 in, 1 out]
                  n153 = Multiply(x=w992, y="Servo 2 Torque Slope") -> (x*y=w993:dbl)
                  n154 = Add(x=w993, y="Servo 2 Torque Intercept") -> (x+y=w991:dbl)
                  "Torq2 number" <- w991
                }
              }
            }
            frame "read3T" {
              n155 = Equal?(x=w1034, y="y") -> (x = y?=w1035:bool)
              n156 = case shown="True" w1035 {
                tunnel: [w1047 0] -> w1010
                tunnel: w1009 -> [w1041 w1053]
                tunnel: w1013 -> [w1045 w1055]
                tunnel: [w1044 w1055] -> w1012
                tunnel: w1034 -> [w1043 _]
                tunnel: [w1040 54] -> w1037
                tunnel: w1036 -> [w1040 _]
                tunnel: [w1039 w1051] -> w1016
                tunnel: w1021 -> [w1039 _]
                frame False {
                  n157 = String To Byte Array(string=w1043) -> (unsigned byte array=w1042:u8[])
                  n158 = Insert Into Array(array=w1045, index=w1041, new element=w1042) -> (w1044:dbl[])
                  n159 = Add(x=w1041, y=1) -> (x+y=w1047:i32)
                }
                frame True {
                  # "Go to read4T"
                  n160 = Byte Array To String(unsigned byte array=w1055) -> (string=w1056:string)
                  n161 = String Subset(string=w1056, offset (0)=0, length (rest)=w1053) -> (substring=w1054:string)
                  n162 = Fract/Exp String To Number(string=w1054) -> (number=w1050:dbl)  [unwired: 3 in, 1 out]
                  n163 = Multiply(x=w1050, y="Servo 3 Torque Slope") -> (x*y=w1052:dbl)
                  n164 = Add(x=w1052, y="Servo 3 Torque Intercept") -> (x+y=w1051:dbl)
                  "Torq3 number" <- w1051
                }
              }
            }
            frame "read4T" {
              n165 = Equal?(x=w1093, y="z") -> (x = y?=w1094:bool)
              n166 = case shown="True" w1094 {
                tunnel: [w1106 0] -> w1066
                tunnel: w1065 -> [w1100 w1112]
                tunnel: w1071 -> [w1104 w1114]
                tunnel: [w1103 w1114] -> w1072
                tunnel: w1093 -> [w1102 _]
                tunnel: [w1099 60] -> w1096
                tunnel: w1095 -> [w1099 _]
                tunnel: [w1098 w1109] -> w1075
                tunnel: w1079 -> [w1098 _]
                frame False {
                  n167 = String To Byte Array(string=w1102) -> (unsigned byte array=w1101:u8[])
                  n168 = Insert Into Array(array=w1104, index=w1100, new element=w1101) -> (w1103:dbl[])
                  n169 = Add(x=w1100, y=1) -> (x+y=w1106:i32)
                }
                frame True {
                  # "Go to read5T"
                  n170 = Byte Array To String(unsigned byte array=w1114) -> (string=w1115:string)
                  n171 = String Subset(string=w1115, offset (0)=0, length (rest)=w1112) -> (substring=w1113:string)
                  n172 = Fract/Exp String To Number(string=w1113) -> (number=w1110:dbl)  [unwired: 3 in, 1 out]
                  n173 = Multiply(x=w1110, y="Servo 4 Torque Slope") -> (x*y=w1111:dbl)
                  n174 = Add(x=w1111, y="Servo 4 Torque Intercept") -> (x+y=w1109:dbl)
                  "Torq4 number" <- w1109
                }
              }
            }
            frame "read5T" {
              n175 = Equal?(x=w1152, y="!") -> (x = y?=w1153:bool)
              n176 = case shown="True" w1153 {
                tunnel: [w1165 0] -> w1128
                tunnel: w1127 -> [w1159 w1171]
                tunnel: w1130 -> [w1163 w1173]
                tunnel: [w1162 w1173] -> w1131
                tunnel: w1152 -> [w1161 _]
                tunnel: [w1158 0] -> w1155
                tunnel: w1154 -> [w1158 _]
                tunnel: [w1157 w1166] -> w1137
                tunnel: w1138 -> [w1157 _]
                frame False {
                  n177 = String To Byte Array(string=w1161) -> (unsigned byte array=w1160:u8[])
                  n178 = Insert Into Array(array=w1163, index=w1159, new element=w1160) -> (w1162:dbl[])
                  n179 = Add(x=w1159, y=1) -> (x+y=w1165:i32)
                }
                frame True {
                  # "Go to none11"
                  n180 = Byte Array To String(unsigned byte array=w1173) -> (string=w1174:string)
                  n181 = String Subset(string=w1174, offset (0)=0, length (rest)=w1171) -> (substring=w1172:string)
                  n182 = Fract/Exp String To Number(string=w1172) -> (number=w1169:dbl)  [unwired: 3 in, 1 out]
                  n183 = Multiply(x=w1169, y="Servo 5 Torque Slope") -> (x*y=w1170:dbl)
                  n184 = Add(x=w1170, y="Servo 5 Torque Intercept") -> (x+y=w1166:dbl)
                  "Torq5 number" <- w1166
                }
              }
            }
          }
        }
      }
    }
    n185 = call-poly <vilib>:"Mean.vi"("X"=w88) -> ("mean"=w43:dbl)  [unwired: 1 out]
    "Calculated Time Delay" <- w43
    n186 = Bundle(0, "mean"=w43, w340) -> (→"Bytes at port":cluster{i32, "mean":dbl, dbl[]})  [unwired: 1 in]
    n187 = Subtract(x=w68, y=1) -> (x-y=w283:i32)
    n188 = Subtract(x=w68, y=1) -> (x-y=w272:i32)
    n189 = Subtract(x=w68, y=1) -> (x-y=w275:i32)
    n190 = Subtract(x=w68, y=1) -> (x-y=w266:i32)
    n191 = Subtract(x=w68, y=1) -> (x-y=w269:i32)
    n192 = Divide(x=1, y=w43) -> (x/y=→"Calculated Sample Frequency":dbl)
    n193 = Index Array(array=w270, index=w272) -> (element=w254:dbl)
    n194 = Index Array(array=w273, index=w275) -> (element=w259:dbl)
    n195 = Index Array(array=w267, index=w269) -> (element=w248:dbl)
    n196 = Index Array(array=w237, index=w266) -> (element=w239:dbl)
    n197 = Index Array(array=w281, index=w283) -> (element=w278:dbl)
    n198 = Less?(x=w242, y="Lowest Servo Angle") -> (x < y?=w243:bool)
    n199 = Greater?(x=w242, y="Highest Servo Angle") -> (0:w245:bool)
    n200 = Or(x=w245, y=w243) -> (x .or. y?=w244:bool)
    n201 = case shown="True" w244 {
      tunnel: w239 -> [_ w417]
      tunnel: w242 -> [w415 _]
      tunnel: [w415 w417] -> w238
      tunnel: [FALSE TRUE] -> w189
      frame False {
      }
      frame True {
      }
    }
    n202 = Greater?(x=w246, y="Highest Servo Angle") -> (0:w249:bool)
    n203 = Less?(x=w246, y="Lowest Servo Angle") -> (x < y?=w250:bool)
    n204 = Or(x=w249, y=w250) -> (x .or. y?=w251:bool)
    n205 = case shown="True" w251 {
      tunnel: w248 -> [_ w421]
      tunnel: w246 -> [w419 _]
      tunnel: [w419 w421] -> w247
      tunnel: [FALSE TRUE] -> w190
      frame False {
      }
      frame True {
      }
    }
    n206 = Or(x=w190, y=w189) -> (x .or. y?=w187:bool)
    n207 = Greater?(x=w252, y="Highest Servo Angle") -> (0:w257:bool)
    n208 = Less?(x=w252, y="Lowest Servo Angle") -> (x < y?=w255:bool)
    n209 = Or(x=w257, y=w255) -> (x .or. y?=w256:bool)
    n210 = case shown="True" w256 {
      tunnel: w254 -> [_ w425]
      tunnel: w252 -> [w423 _]
      tunnel: [w423 w425] -> w253
      tunnel: [FALSE TRUE] -> w188
      frame False {
      }
      frame True {
      }
    }
    n211 = Or(x=w188, y=w187) -> (x .or. y?=w185:bool)
    n212 = Greater?(x=w258, y="Highest Servo Angle") -> (0:w263:bool)
    n213 = Less?(x=w258, y="Lowest Servo Angle") -> (x < y?=w261:bool)
    n214 = Or(x=w263, y=w261) -> (x .or. y?=w262:bool)
    n215 = case shown="True" w262 {
      tunnel: w259 -> [_ w429]
      tunnel: w258 -> [w427 _]
      tunnel: [w427 w429] -> w260
      tunnel: [FALSE TRUE] -> w186
      frame False {
      }
      frame True {
      }
    }
    n216 = Or(x=w186, y=w185) -> (x .or. y?=w183:bool)
    n217 = Less?(x=w276, y="Lowest Servo Angle") -> (x < y?=w277:bool)
    n218 = Greater?(x=w276, y="Highest Servo Angle") -> (0:w280:bool)
    n219 = Or(x=w280, y=w277) -> (x .or. y?=w279:bool)
    n220 = case shown="True" w279 {
      tunnel: w278 -> [_ w433]
      tunnel: w276 -> [w431 _]
      tunnel: [w431 w433] -> w264
      tunnel: [FALSE TRUE] -> w184
      frame False {
      }
      frame True {
      }
    }
    n221 = Or(x=w184, y=w183) -> (x .or. y?=→"Minimum or Maximum Angle Exceeded":bool)
    n222 = Insert Into Array(array=w281, index=w68, new element=w264) -> (w70:dbl[])
    n223 = Insert Into Array(array=w273, index=w68, new element=w260) -> (w72:dbl[])
    n224 = Insert Into Array(array=w237, index=w68, new element=w238) -> (w86:dbl[])
    n225 = Insert Into Array(array=w270, index=w68, new element=w253) -> (w76:dbl[])
    n226 = Insert Into Array(array=w267, index=w68, new element=w247) -> (w80:dbl[])
    n227 = Greater?(x=w169, y="Max Torque") -> (0:w163:bool)
    n228 = Greater?(x=w165, y="Max Torque") -> (0:w162:bool)
    n229 = Greater?(x=w166, y="Max Torque") -> (0:w161:bool)
    n230 = Or(x=w162, y=w163) -> (x .or. y?=w160:bool)
    n231 = Greater?(x=w167, y="Max Torque") -> (0:w159:bool)
    n232 = Subtract(x=w137, y=w141) -> (x-y=w142:dbl)
    n233 = Subtract(x=w138, y=w141) -> (x-y=w143:dbl)
    n234 = Or(x=w161, y=w160) -> (x .or. y?=w156:bool)
    n235 = Greater?(x=w168, y="Max Torque") -> (0:w158:bool)
    n236 = Subtract(x=w136, y=w141) -> (x-y=w144:dbl)
    n237 = Subtract(x=w139, y=w141) -> (x-y=w145:dbl)
    n238 = Or(x=w159, y=w156) -> (x .or. y?=w157:bool)
    n239 = Subtract(x=w140, y=w141) -> (x-y=w146:dbl)
    n240 = Insert Into Array(array=w292, index=w68, new element=w169) -> (w181:dbl[])
    n241 = Insert Into Array(array=w291, index=w68, new element=w165) -> (w179:dbl[])
    n242 = Insert Into Array(array=w288, index=w68, new element=w168) -> (w180:dbl[])
    n243 = Or(x=w158, y=w157) -> (x .or. y?=→"Maximum Torque Exceeded":bool)
    n244 = Insert Into Array(array=w290, index=w68, new element=w166) -> (w178:dbl[])
    n245 = Insert Into Array(array=w289, index=w68, new element=w167) -> (w177:dbl[])
    n246 = Build Array(w146, w145, w144, w143, w142) -> (w111:dbl[])
    "Output Angles" <- w111
    n247 = call "PlotSubArray.vi"("Time Step (s)"=w43, "Plot Last x Seconds"="Plot Last x Seconds", "Iteration"=w68, "Array"=w80) -> ("Sub Array"=w61:dbl[], "Time Offset"=w78:dbl)  [unwired: 6 in]
    n248 = call "PlotSubArray.vi"("Time Step (s)"=w43, "Plot Last x Seconds"="Plot Last x Seconds", "Iteration"=w68, "Array"=w71) -> ("Sub Array"=w67:dbl[])  [unwired: 6 in, 1 out]
    n249 = call "PlotSubArray.vi"("Time Step (s)"=w43, "Plot Last x Seconds"="Plot Last x Seconds", "Iteration"=w68, "Array"=w79) -> ("Sub Array"=w60:dbl[])  [unwired: 6 in, 1 out]
    n250 = call "PlotSubArray.vi"("Time Step (s)"=w43, "Plot Last x Seconds"="Plot Last x Seconds", "Iteration"=w68, "Array"=w72) -> ("Sub Array"=w65:dbl[], "Time Offset"=w74:dbl)  [unwired: 6 in]
    n251 = call "PlotSubArray.vi"("Time Step (s)"=w43, "Plot Last x Seconds"="Plot Last x Seconds", "Iteration"=w68, "Array"=w73) -> ("Sub Array"=w64:dbl[])  [unwired: 6 in, 1 out]
    n252 = call "PlotSubArray.vi"("Time Step (s)"=w43, "Plot Last x Seconds"="Plot Last x Seconds", "Iteration"=w68, "Array"=w77) -> ("Sub Array"=w63:dbl[])  [unwired: 6 in, 1 out]
    n253 = call "PlotSubArray.vi"("Time Step (s)"=w43, "Plot Last x Seconds"="Plot Last x Seconds", "Iteration"=w68, "Array"=w76) -> ("Sub Array"=w62:dbl[], "Time Offset"=w75:dbl)  [unwired: 6 in]
    n254 = call "PlotSubArray.vi"("Time Step (s)"=w43, "Plot Last x Seconds"="Plot Last x Seconds", "Iteration"=w68, "Array"=w87) -> ("Sub Array"=w58:dbl[])  [unwired: 6 in, 1 out]
    n255 = call "PlotSubArray.vi"("Time Step (s)"=w43, "Plot Last x Seconds"="Plot Last x Seconds", "Iteration"=w68, "Array"=w86) -> ("Sub Array"=w59:dbl[], "Time Offset"=w85:dbl)  [unwired: 6 in]
    n256 = call "PlotSubArray.vi"("Time Step (s)"=w43, "Plot Last x Seconds"="Plot Last x Seconds", "Iteration"=w68, "Array"=w70) -> ("Sub Array"=w66:dbl[], "Time Offset"=w69:dbl)  [unwired: 6 in]
    n257 = Divide(x="Length of Segments", y=100) -> (x/y=w122:dbl)
    n258 = Initialize Array(0.0 ("element"), 1 ("dimension size")) -> (w149:dbl[])
    n259 = Initialize Array(0.0 ("element"), 1 ("dimension size")) -> (w148:dbl[])
    n260 = Build Array(w63, w62) -> (w307:dbl[][])
    n261 = Build Array(w58, w59) -> (w84:dbl[][])
    n262 = Build Array(w60, w61) -> (w82:dbl[][])
    n263 = Build Array(w67, w66) -> (w309:dbl[][])
    n264 = call "PlotSubArray.vi"("Time Step (s)"=w43, "Plot Last x Seconds"="Plot Last x Seconds", "Iteration"=w68, "Array"=w181) -> ("Sub Array"=w176:dbl[], "Time Offset"=w57:dbl)  [unwired: 6 in]
    n265 = Build Array(w64, w65) -> (w308:dbl[][])
    n266 = call "PlotSubArray.vi"("Time Step (s)"=w43, "Plot Last x Seconds"="Plot Last x Seconds", "Iteration"=w68, "Array"=w179) -> ("Sub Array"=w175:dbl[])  [unwired: 6 in, 1 out]
    n267 = call "PlotSubArray.vi"("Time Step (s)"=w43, "Plot Last x Seconds"="Plot Last x Seconds", "Iteration"=w68, "Array"=w178) -> ("Sub Array"=w174:dbl[])  [unwired: 6 in, 1 out]
    n268 = call "PlotSubArray.vi"("Time Step (s)"=w43, "Plot Last x Seconds"="Plot Last x Seconds", "Iteration"=w68, "Array"=w177) -> ("Sub Array"=w173:dbl[])  [unwired: 6 in, 1 out]
    n269 = call "PlotSubArray.vi"("Time Step (s)"=w43, "Plot Last x Seconds"="Plot Last x Seconds", "Iteration"=w68, "Array"=w180) -> ("Sub Array"=w172:dbl[])  [unwired: 6 in, 1 out]
    n270 = Bundle("Time Offset"=w78, "mean"=w43, w82) -> (→"Servo 4 Position":cluster{" Time Offset":dbl, "mean":dbl, dbl[][]})  [unwired: 1 in]
    n271 = Bundle("Time Offset"=w75, "mean"=w43, w307) -> (→"Servo 3 Position":cluster{" Time Offset":dbl, "mean":dbl, dbl[][]})  [unwired: 1 in]
    n272 = Bundle("Time Offset"=w74, "mean"=w43, w308) -> (→"Servo 2 Position":cluster{" Time Offset":dbl, "mean":dbl, dbl[][]})  [unwired: 1 in]
    n273 = Bundle("Time Offset"=w85, "mean"=w43, w84) -> (→"Servo 5 Position":cluster{" Time Offset":dbl, "mean":dbl, dbl[][]})  [unwired: 1 in]
    n274 = Bundle("Time Offset"=w69, "mean"=w43, w309) -> (→"Servo 1 Position":cluster{" Time Offset":dbl, "mean":dbl, dbl[][]})  [unwired: 1 in]
    n275 = Build Array(w176, w175, w174, w173, w172) -> (w171:dbl[][])
    n276 = for {
      N: w93 -> [_]
      shift-right: [w353] -> _
      shift-left: 0.0 -> [w370]
      tunnel: w111 -> [w369]
      shift-right: [w363] -> w118
      shift-left: w149 -> [w351]
      shift-right: [w362] -> w117
      shift-left: w148 -> [w350]
      tunnel: w122 -> [w349]
      i -> [w361]
      (unwired) 100
      # "phi"
      # "L"
      n277 = Index Array(array=w369, index=w361) -> (element=w368:dbl)
      n278 = Index Array(array=w351, index=w361) -> (element=w367:dbl)
      n279 = Index Array(array=w350, index=w361) -> (element=w364:dbl)
      n280 = Divide(x=3.141592653589793, y=180) -> (x/y=w352:dbl)
      n281 = Add(x=w368, y=w370) -> (x+y=w353:dbl)
      n282 = Multiply(x=w352, y=w353) -> (x*y=w355:dbl)
      n283 = Multiply(x=w352, y=w353) -> (x*y=w354:dbl)
      n284 = Increment(x=w361) -> (x+1=w360:i32)
      n285 = Cosine(x=w355) -> (cos(x)=w359:dbl)
      n286 = Sine(x=w354) -> (sin(x)=w358:dbl)
      n287 = Multiply(x=w359, y=w349) -> (x*y=w366:dbl)
      n288 = Multiply(x=w349, y=w358) -> (x*y=w365:dbl)
      n289 = Add(x=w367, y=w366) -> (x+y=w348:dbl)
      n290 = Add(x=w365, y=w364) -> (x+y=w347:dbl)
      n291 = Insert Into Array(array=w351, index=w360, new element=w348) -> (w363:dbl[])
      n292 = Insert Into Array(array=w350, index=w360, new element=w347) -> (w362:dbl[])
    }
    n293 = Bundle("Time Offset"=w57, "mean"=w43, w171) -> (→"Servo Torque":cluster{" Time Offset":dbl, "mean":dbl, dbl[][]})  [unwired: 1 in]
    n294 = Increment(x=w93) -> (x+1=w135:dbl)
    n295 = Increment(x=w93) -> (x+1=w132:dbl)
    n296 = Increment(x=w93) -> (x+1=w119:dbl)
    n297 = Multiply(x=w135, y="Length of Segments") -> (x*y=w133:dbl)
    n298 = Multiply(x=w132, y="Length of Segments") -> (x*y=w129:dbl)
    n299 = Divide(x="Length of Segments", y=5) -> (x/y=w130:dbl)
    n300 = Divide(x="Length of Segments", y=5) -> (x/y=w131:dbl)
    n301 = Multiply(x=-1, y=w133) -> (x*y=w134:dbl)
    n302 = Bundle(w125, w129, w122, w130, w125) -> (w124:cluster{i32, dbl, dbl, dbl, i32})  [unwired: 1 in]
    n303 = for {
      N: w119 -> [_]
      tunnel: w118 -> [w346] mode=indexing
      tunnel: w117 -> [w344] mode=indexing
      tunnel: [w343] -> w115 mode=indexing
      tunnel: [w342] -> w114 mode=indexing
      w345 = 100
      # "Convert nodes from m to cm"
      n304 = Multiply(x=w346, y=w345) -> (x*y=w343:dbl)
      n305 = Multiply(x=w345, y=w344) -> (x*y=w342:dbl)
    }
    n306 = Bundle(w134, w133, w122, w131, w134) -> (w123:cluster{dbl, dbl, dbl, dbl, dbl})  [unwired: 1 in]
    n307 = property on="Waveform" class="XYGraph (strict)"("XScale.Range"=w124) -> ()  [unwired: 2 in, 2 out]
    n308 = property on="Waveform" class="XYGraph (strict)"("YScale.Range"=w123) -> ()  [unwired: 2 in, 2 out]
    n309 = property on="Waveform" class="XYGraph (strict)"("Plot.Point Style"=u8 2) -> ()  [unwired: 2 in, 2 out]
    n310 = Bundle(w115, w114) -> (w113:cluster{dbl[], dbl[]})  [unwired: 1 in]
    n311 = Build Array(w120, w113) -> (→"Waveform":cluster{"X Nodes":dbl[], "Y Nodes":dbl[]}[])
  }
  n312 = VISA Close(VISA resource name=w29, error in (no error)=w28) -> ()  [unwired: 1 out]
  n313 = case shown="True" w30 {
    tunnel: w1 -> [_ w1240]
    tunnel: w27 -> [_ w1239]
    tunnel: w25 -> [_ w1226]
    tunnel: w24 -> [_ w1225]
    tunnel: w23 -> [_ w1224]
    tunnel: w22 -> [_ w1223]
    tunnel: w21 -> [_ w1214]
    tunnel: w20 -> [_ w1213]
    tunnel: w19 -> [_ w1212]
    tunnel: w18 -> [_ w1211]
    tunnel: w17 -> [_ w1209]
    tunnel: w16 -> [_ w1199]
    tunnel: w15 -> [_ w1198]
    tunnel: w14 -> [_ w1197]
    tunnel: w13 -> [_ w1196]
    frame False {
    }
    frame True {
      n314 = call "Convert to Dynamic Data9"("Array"=w1223) -> ("Dynamic Data Type"=w1228:dynamicdata)  [unwired: 3 in]
      n315 = call "Convert to Dynamic Data11"("Array"=w1213) -> ("Dynamic Data Type"=w1220:dynamicdata)  [unwired: 3 in]
      n316 = call "Convert to Dynamic Data13"("Array"=w1211) -> ("Dynamic Data Type"=w1216:dynamicdata)  [unwired: 3 in]
      n317 = call "Convert to Dynamic Data"("Array"=w1239) -> ("Dynamic Data Type"=w1238:dynamicdata)  [unwired: 3 in]
      n318 = call "Convert to Dynamic Data12"("Array"=w1212) -> ("Dynamic Data Type"=w1218:dynamicdata)  [unwired: 3 in]
      n319 = call "Convert to Dynamic Data10"("Array"=w1214) -> ("Dynamic Data Type"=w1222:dynamicdata)  [unwired: 3 in]
      n320 = call "Convert to Dynamic Data17"("Array"=w1197) -> ("Dynamic Data Type"=w1202:dynamicdata)  [unwired: 3 in]
      n321 = call "Convert to Dynamic Data18"("Array"=w1196) -> ("Dynamic Data Type"=w1200:dynamicdata)  [unwired: 3 in]
      n322 = call "Convert to Dynamic Data16"("Array"=w1198) -> ("Dynamic Data Type"=w1204:dynamicdata)  [unwired: 3 in]
      n323 = call "Convert to Dynamic Data15"("Array"=w1199) -> ("Dynamic Data Type"=w1206:dynamicdata)  [unwired: 3 in]
      n324 = call "Convert to Dynamic Data14"("Array"=w1209) -> ("Dynamic Data Type"=w1208:dynamicdata)  [unwired: 3 in]
      n325 = call "Convert to Dynamic Data2"("Array"=w1240) -> ("Dynamic Data Type"=w1237:dynamicdata)  [unwired: 3 in]
      n326 = call "Convert to Dynamic Data6"("Array"=w1226) -> ("Dynamic Data Type"=w1234:dynamicdata)  [unwired: 3 in]
      n327 = call "Convert to Dynamic Data8"("Array"=w1224) -> ("Dynamic Data Type"=w1230:dynamicdata)  [unwired: 3 in]
      n328 = call "Convert to Dynamic Data7"("Array"=w1225) -> ("Dynamic Data Type"=w1232:dynamicdata)  [unwired: 3 in]
      n329 = xnode "Set Dynamic Data Attributes"("Signals In"=w1237, "Signal Name"="Servo 1 Commanded Position") -> ("Signals Out"=w1195:dynamicdata)  [unwired: 2 in, 1 out]
      n330 = xnode "Set Dynamic Data Attributes"("Signals In"=w1234, "Signal Name"="Servo 2 Commanded Position") -> ("Signals Out"=w1194:dynamicdata)  [unwired: 2 in, 1 out]
      n331 = xnode "Set Dynamic Data Attributes"("Signals In"=w1230, "Signal Name"="Servo 4 Commanded Position") -> ("Signals Out"=w1192:dynamicdata)  [unwired: 2 in, 1 out]
      n332 = xnode "Set Dynamic Data Attributes"("Signals In"=w1232, "Signal Name"="Servo 3 Commanded Position") -> ("Signals Out"=w1193:dynamicdata)  [unwired: 2 in, 1 out]
      n333 = xnode "Set Dynamic Data Attributes"("Signals In"=w1228, "Signal Name"="Servo 5 Commanded Position") -> ("Signals Out"=w1191:dynamicdata)  [unwired: 2 in, 1 out]
      n334 = xnode "Set Dynamic Data Attributes"("Signals In"=w1238, "Signal Name"="Servo 1 Feedback Position") -> ("Signals Out"=w1190:dynamicdata)  [unwired: 2 in, 1 out]
      n335 = xnode "Set Dynamic Data Attributes"("Signals In"=w1218, "Signal Name"="Servo 1 Feedback Position") -> ("Signals Out"=w1187:dynamicdata)  [unwired: 2 in, 1 out]
      n336 = xnode "Set Dynamic Data Attributes"("Signals In"=w1220, "Signal Name"="Servo 1 Feedback Position") -> ("Signals Out"=w1188:dynamicdata)  [unwired: 2 in, 1 out]
      n337 = xnode "Set Dynamic Data Attributes"("Signals In"=w1202, "Signal Name"="Servo 4  Torque") -> ("Signals Out"=w1182:dynamicdata)  [unwired: 2 in, 1 out]
      n338 = xnode "Set Dynamic Data Attributes"("Signals In"=w1200, "Signal Name"="Servo 5  Torque") -> ("Signals Out"=w1181:dynamicdata)  [unwired: 2 in, 1 out]
      n339 = xnode "Set Dynamic Data Attributes"("Signals In"=w1222, "Signal Name"="Servo 1 Feedback Position") -> ("Signals Out"=w1189:dynamicdata)  [unwired: 2 in, 1 out]
      n340 = xnode "Set Dynamic Data Attributes"("Signals In"=w1204, "Signal Name"="Servo 3  Torque") -> ("Signals Out"=w1183:dynamicdata)  [unwired: 2 in, 1 out]
      n341 = xnode "Set Dynamic Data Attributes"("Signals In"=w1216, "Signal Name"="Servo 1 Feedback Position") -> ("Signals Out"=w1186:dynamicdata)  [unwired: 2 in, 1 out]
      n342 = xnode "Set Dynamic Data Attributes"("Signals In"=w1206, "Signal Name"="Servo 2  Torque") -> ("Signals Out"=w1184:dynamicdata)  [unwired: 2 in, 1 out]
      n343 = xnode "Set Dynamic Data Attributes"("Signals In"=w1208, "Signal Name"="Servo 1  Torque") -> ("Signals Out"=w1185:dynamicdata)  [unwired: 2 in, 1 out]
      n344 = Merge Signals(w1195, w1194, w1193, w1192, w1191, w1190, w1189, w1188, w1187, w1186, w1185, w1184, w1183, w1182, w1181) -> (w1180:dynamicdata)
      n345 = call "Write To Measurement File"("Signals"=w1180, "Filename"="Filename", "Comment"="Comment") -> ()  [unwired: 14 in, 3 out]
    }
  }
